vi "ZPL Config OVP.vi"(6 "Settle (1 mS)":u32=1, 8 "error":errorcluster, 10 "OVP":dbl format="%.4f", 11 "VISA":refnum<visa-resource-name>) -> (0 "error out":errorcluster, 3 "VISA out":refnum<visa-resource-name>)   [LabVIEW 2015]
doc: "This command sets the over voltage protection (OVP) level of the power supply.\n\nThis VI will wait for \"Settle\" milliseconds after setting the limit to allow the output to reach the new setting. If unwired, there will be no delay"
panel:
  # "Lambda ZPLUS \n Serial Port\n  DC Power Supplies"
  # "Set the OVP"
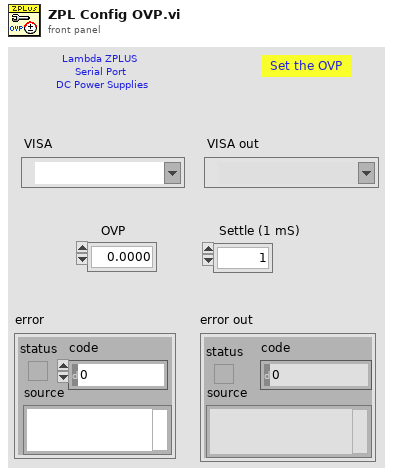
[diagram p1: front panel]
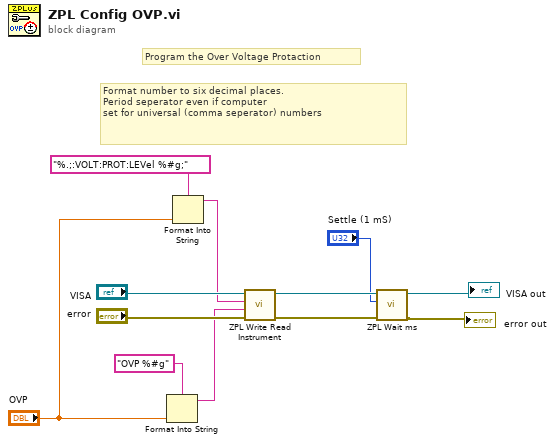
[diagram p0: block diagram]
diagram:
  # "Format number to six decimal places.\nPeriod seperator even if computer \nset for universal (comma seperator) numbers"
  # "Program the Over Voltage Protaction"
  n1 = Format Into String(format string="OVP %#g", "OVP") -> (resulting string=w7:string)  [unwired: 2 in, 1 out]
  n2 = Format Into String(format string="%.;:VOLT:PROT:LEVel %#g;", "OVP") -> (resulting string=w10:string)  [unwired: 2 in, 1 out]
  n3 = call "ZPL Write Read Instrument.vi"("error in"="error", "Write Command/Query GEN"=w7, "Write Command/Query SCPI"=w10, "VISA"="VISA") -> ("error out"=w4:errorcluster, "VISA  out"=w5:refnum<visa-resource-name>)  [unwired: 5 in, 1 out]
  n4 = call "ZPL Wait ms.vi"("error"=w4, "Delay (1 mS)"="Settle (1 mS)", "VISA"=w5) -> ("error out"=→"error out":errorcluster, "VISA out"=→"VISA out":refnum<visa-resource-name>)  [unwired: 7 in]
